vi "Emergency Stop.vi"(8 "error in (no error)":errorcluster, 10 "Wheel (-1: all)":i32, 11 "Filter Wheel Simulator in":refnum<class "Filter Wheel Simulator.lvclass">) -> (0 "error out":errorcluster, 3 "Filter Wheel Simulator out":refnum<class "Filter Wheel Simulator.lvclass">)   [LabVIEW 2021, in "Filter Wheel Simulator.lvclass"]
uses:
  Filter Wheel Simulator.lvclass
  Filter Wheel Simulator.lvclass/Filter Wheel Simulator.ctl
  Filter Wheel Object/Filter Wheel.lvclass
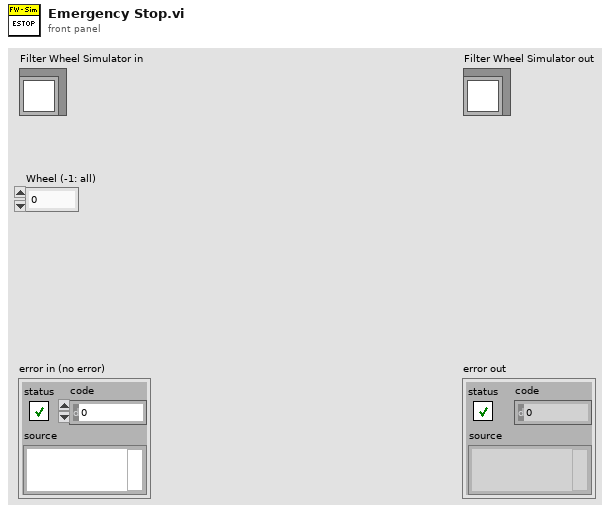
[diagram p1: front panel]
types:
  T1 = typedef "Filter Wheel Simulator.lvclass/Filter Wheel cluster Simulated Status.ctl" = cluster{"Move Start Time":timestamp, "Moving?":bool, "Target Pos":dbl, "Direction":bool}
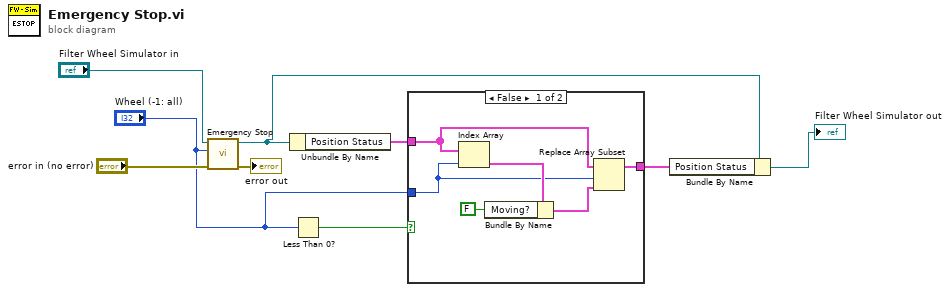
[diagram p0: block diagram]
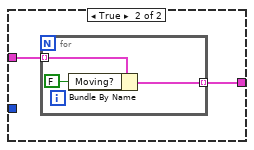
[diagram p2: hidden frame]
diagram:
  n1 = call-parent "Emergency Stop.vi"("error in (no error)"="error in (no error)", "Wheel (-1: all)"="Wheel (-1: all)", "Filter Wheel in"="Filter Wheel Simulator in") -> ("error out"=→"error out":errorcluster, "Filter Wheel out"=w1:refnum<class "Filter Wheel Simulator.lvclass">)  [unwired: 7 in]
  n2 = Unbundle By Name(w1) -> ("Position Status"=w6:T1[])
  n3 = Less Than 0?(x="Wheel (-1: all)") -> (x < 0?=w3:bool)
  n4 = case shown="False" w3 {
    tunnel: w6 -> [w11 w17]
    tunnel: [w10 w16] -> w5
    tunnel: "Wheel (-1: all)" -> [w12 _]
    frame False {
      n5 = Index Array(array=w11, index=w12) -> (element=w15:T1)
      n6 = Bundle By Name(cluster=w15, "Moving?"=FALSE) -> (w13:T1)
      n7 = Replace Array Subset(array=w11, new element=w13, index=w12) -> (w10:T1[])
    }
    frame True {
      n8 = for {
        tunnel: w17 -> [w20] mode=indexing
        tunnel: [w18] -> w16 mode=indexing
        n9 = Bundle By Name(cluster=w20, "Moving?"=FALSE) -> (w18:T1)
      }
    }
  }
  n10 = Bundle By Name(cluster=w1, "Position Status"=w5) -> (→"Filter Wheel Simulator out":refnum<class "Filter Wheel Simulator.lvclass">)
